vi "rx.vi"(0 "HW parameters In":T5={"Device IP Address"="192.168.11.6", "Active Antenna"="RX1", "Carrier Frequency (Hz)"=915000000.0, "Gain (dB)"=10.0, "Trigger Level"=0.01, "Bandwidth (Hz)"=40000000.0, "Reference Position (%)"=10.0, "Capture Time (s)"=0.0004, "Simulate"=FALSE} {"Capture Time (s)" format="%.2p"; "Bandwidth (Hz)" format="%.2p"; "Trigger Level" format="%#.3p"; "Gain (dB)" format="%.2f"; "Carrier Frequency (Hz)" format="%.2p"}, 2 "Modulation Parameters In":T1 {"RX Parameters"."RX Sample Rate" items=["4M"]}, 4 "Queues In":T4, 5 "Received IQ\nwaveform":cluster{"t0":dbl, "dt":dbl, "Y":cdb[]} {"Y" format="%.2g"; "dt" format="%.2g"; "t0" format="%.2g"}, 7 "error in (no error)":errorcluster) -> (8 "overhead offset":i32, 9 "key bit sequence":u8[](array[numeric]), 10 "symbol rate":dbl format="%#_6p", 11 "offset":i32, 12 "bit-error rate":dbl, 13 "Received IQ Graph":cluster{dbl[], dbl[]}(graph) caption="IQ Graph", 14 "Received Magnitude":dbl[](graph), 15 "Received Constellation Graph":T3(graph) caption="Constellation Graph", 17 "Received Eye Diagram":cluster{"t0":dbl, "dt":dbl, "Y":dbl[]}[](graph) caption="Eye Diagram", 18 "Received Phase":dbl[](graph), 19 "Received Power Spectrum Density":dbl[](graph), 20 "HW parameters Out":T5={"Device IP Address"="192.168.11.6", "Active Antenna"="RX1", "Carrier Frequency (Hz)"=915000000.0, "Gain (dB)"=10.0, "Trigger Level"=0.01, "Bandwidth (Hz)"=40000000.0, "Reference Position (%)"=10.0, "Capture Time (s)"=0.0004, "Simulate"=FALSE} {"Capture Time (s)" format="%.2p"; "Bandwidth (Hz)" format="%.2p"; "Trigger Level" format="%#.3p"; "Gain (dB)" format="%.2f"; "Carrier Frequency (Hz)" format="%.2p"}, 22 "Modulation Parameters Out":T1 {"RX Parameters"."RX Sample Rate" items=["4M"]}, 24 "Queues  Out":T4, 26 "Measured channel impairements":T6, 27 "error out":errorcluster)   [LabVIEW 2012]
uses:
  EE 497/LABS/SDR/control_type_defs.llb/rx_hw params.ctl
  EE 497/LABS/SDR/control_type_defs.llb/Queues.ctl
panel:
  in  "RX Graphs":T2(tab)
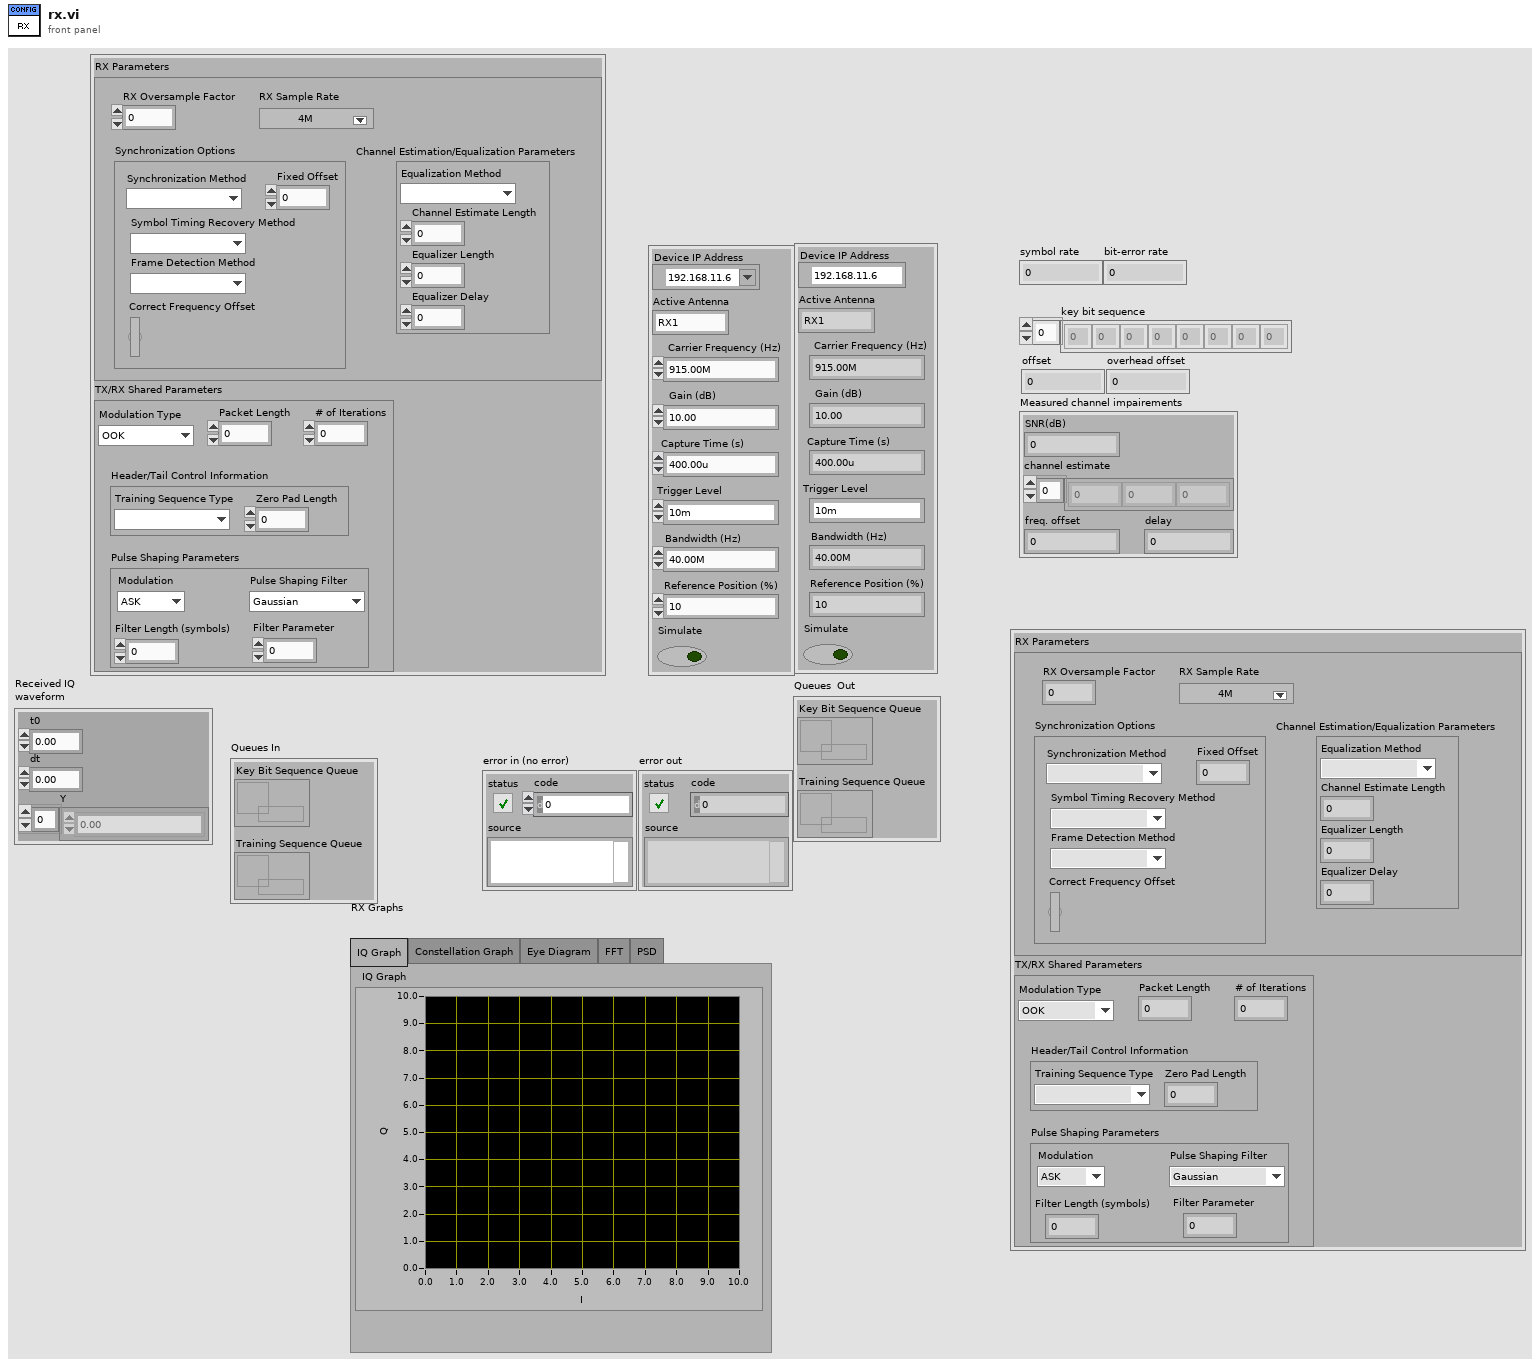
[diagram p1: front panel]
types:
  T1 = cluster{"RX Parameters":cluster{"RX Oversample Factor":dbl, "RX Sample Rate":dbl, "Synchronization Options":cluster{"Synchronization Method":enum16{""}, "Symbol Timing Recovery Method ":enum16{""}, "Fixed Offset":dbl, "Frame Detection Method":enum16{""}, "Correct Frequency Offset":bool}, "Channel Estimation/Equalization Parameters":cluster{"Equalization Method":enum16{""}, "Channel Estimate Length":dbl, "Equalizer Length":dbl, "Equalizer Delay":dbl}}, "TX/RX Shared Parameters":cluster{"Modulation Type":enum16{"OOK", "FSK"}, "Packet Length":dbl, "# of Iterations":dbl, "Pulse Shaping Parameters":cluster{"Modulation":enum16{"ASK", "FSK", "PSK", "QAM", "MSK", "PAM"}, "Pulse Shaping Filter":enum16{"Gaussian"}, "Filter Length (symbols)":dbl, "Filter Parameter":dbl}, "Header/Tail Control Information":cluster{"Training Sequence Type":enum16{""}, "Zero Pad Length":dbl}}}
  T2 = enum32{"IQ Graph", "Constellation Graph", "Eye Diagram", "FFT", "PSD"}
  T3 = cluster{"Decimated Array":dbl[], "Decimated Array":dbl[]}[]
  T4 = typedef "Queues.ctl" = cluster{"Key Bit Sequence Queue":refnum<queue>, "Training Sequence Queue":refnum<queue>}
  T5 = typedef "rx_hw params.ctl" = cluster{"Device IP Address":refnum<k15>, "Active Antenna":string, "Carrier Frequency (Hz)":dbl, "Gain (dB)":dbl, "Trigger Level":dbl, "Bandwidth (Hz)":dbl, "Reference Position (%)":dbl, "Capture Time (s)":dbl, "Simulate":bool}
  T6 = cluster{"SNR(dB)":dbl, "channel estimate":cdb[], "freq. offset":dbl, "delay":dbl}
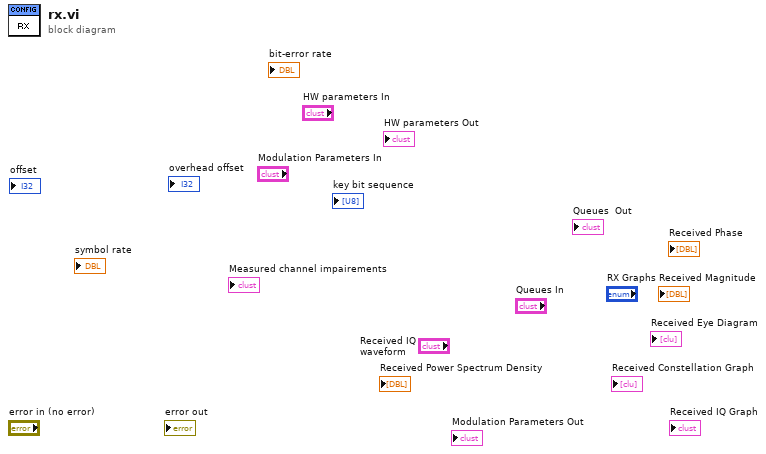
[diagram p0: block diagram]
diagram:
